vi "Test LCR-meter.vi"() -> ()   [LabVIEW 2020, in "LCR Meter.lvclass"]
uses:
  LCR Meter.lvclass
  Agilent 428x/Agilent 428x.lvclass
  C:/Sandbox/RF Bench/Source Code/WiSpry Test Framework/Instruments/Instrument.lvclass
  Instrument.lvclass/Instrument.ctl
  Instrument.lvclass
panel:
  in  "result":path
  in  "Delay Time (s)":dbl=1.0
  in  "Stop Button":bool
  in  "VISA resource name":refnum<visa-resource-name>
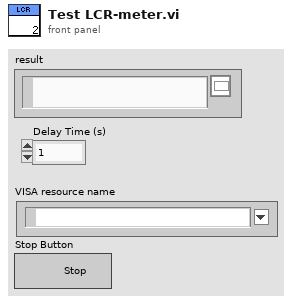
[diagram p1: front panel]
types:
  T1 = enum16{"open", "replace", "create", "open or create", "replace or create", "replace or create with confirmation"}
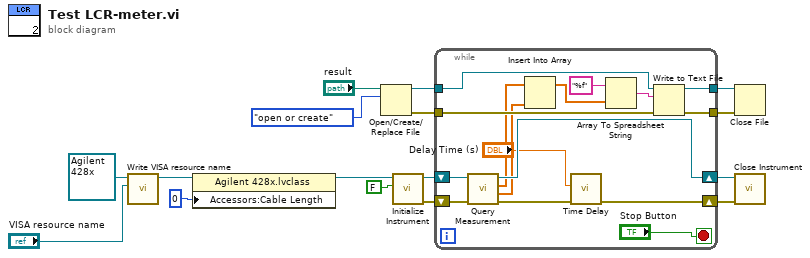
[diagram p0: block diagram]
diagram:
  n1 = call "Write VISA resource name.vi"("VISA resource name"="VISA resource name", "Instrument in"=refnum<class "Agilent 428x.lvclass"> refnum ("Agilent 428x.lvclass")) -> ("Instrument out"=w3:refnum<class "Agilent 428x.lvclass">)  [unwired: 9 in]
  n2 = property class="Agilent 428x.lvclass"(reference=w3, "Accessors:Cable Length"=u32 0 ("Cable Length")) -> (reference out=w2:refnum<class "Agilent 428x.lvclass">)  [unwired: 1 in, 1 out]
  n3 = Open/Create/Replace File(file path (use dialog)="result", operation (0:open)=T1."open or create") -> (refnum out=w11:refnum<file>, error out=w10:errorcluster)  [unwired: 4 in, 1 out]
  n4 = call-dynamic "Initialize Instrument.vi"("Reset"=FALSE, "Agilent 428x in"=w2) -> ("error out"=w14:errorcluster, "Agilent 428x out"=w15:refnum<class "Agilent 428x.lvclass">)  [unwired: 8 in]
  n5 = while {
    shift-right: [w30] -> w13
    shift-left: w15 -> [w32]
    shift-right: [w18] -> w12
    shift-left: w14 -> [w31]
    tunnel: w11 -> [w26]
    tunnel: w10 -> [w25]
    tunnel: [w24] -> w9
    tunnel: [w23] -> w8
    stop <- "Stop Button" stop-if-true
    n6 = call-dynamic "Query Measurement.vi"("error in (no error)"=w31, "Agilent 428x in"=w32) -> ("error out"=w27:errorcluster, "Secondary results"=w17:dbl[], "Capacitances (fF)"=w22:dbl[], "Agilent 428x out"=w30:refnum<class "Agilent 428x.lvclass">)  [unwired: 6 in]
    n7 = Insert Into Array(array=w22, new element=w17) -> (w21:dbl[])  [unwired: 1 in]
    n8 = call "Time Delay"("error in (no error)"=w27, "Delay Time (s)"="Delay Time (s)") -> ("error out"=w18:errorcluster)  [unwired: 9 in]
    n9 = Array To Spreadsheet String(array=w21, 3:"%f" ("format string")) -> (spreadsheet string=w20:string)  [unwired: 1 in]
    n10 = Write to Text File(file (use dialog)=w26, text=w20, error in=w25) -> (refnum out=w24:refnum<file>, error out=w23:errorcluster)  [unwired: 1 in, 1 out]
  }
  n11 = Close File(refnum=w9, error in=w8) -> ()  [unwired: 2 out]
  n12 = call-dynamic "Close Instrument.vi"("error in (no error)"=w12, "Instrument in"=w13) -> ()  [unwired: 8 in, 2 out]
